vi "backup HPLC file.vi"(8 "error in (no error)":errorcluster, 10 "Backup location":path, 11 "HPLC":path) -> (0 "error out":errorcluster)   [LabVIEW 2017]
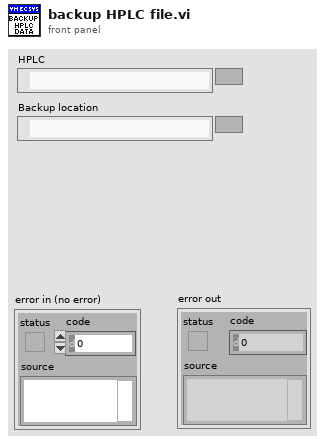
[diagram p1: front panel]
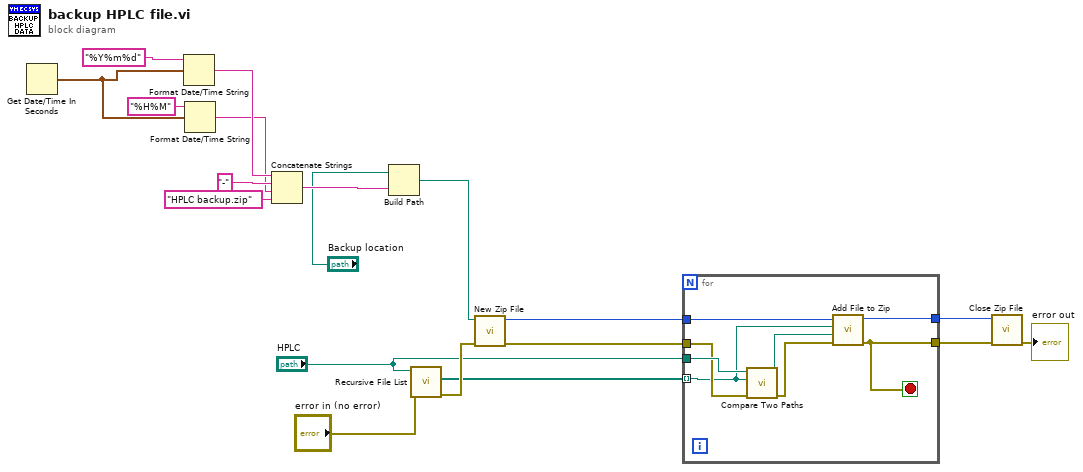
[diagram p0: block diagram]
diagram:
  n1 = Get Date/Time In Seconds() -> (seconds since 1Jan1904=w18:timestamp)
  n2 = Format Date/Time String(time format string (%c)="%Y%m%d", seconds (now)=w18) -> (date/time string=w16:string)  [unwired: 1 in]
  n3 = Format Date/Time String(time format string (%c)="%H%M", seconds (now)=w18) -> (date/time string=w14:string)  [unwired: 1 in]
  n4 = Concatenate Strings(w16, "-" ("string"), w14, "HPLC backup.zip" ("string")) -> (w13:string)
  n5 = Build Path(base path="Backup location", name or relative path=w13) -> (appended path=w1:path)
  n6 = call <vilib>:"Recursive File List.vi"("error in (no error)"="error in (no error)", "Folder Path"="HPLC") -> ("error out"=w12:errorcluster, "All Files in Dir"=w11:path[])  [unwired: 5 in, 3 out]
  n7 = call <vilib>:"New Zip File.vi"("error in (no error)"=w12, "target"=w1) -> ("error out"=w10:errorcluster, "zip file out"=w9:i64)  [unwired: 3 in, 1 out]
  n8 = for {
    tunnel: w11 -> [w23] mode=indexing
    tunnel: "HPLC" -> [w27]
    tunnel: w10 -> [w25]
    tunnel: w9 -> [w24]
    tunnel: [w21] -> w8
    tunnel: [w20] -> w7
    stop <- w20 stop-if-true
    n9 = call <vilib>:"Compare Two Paths.vi"("error in (no error)"=w25, "Path 2"=w23, "Path 1"=w27) -> ("error out"=w26:errorcluster, "Relative Path from 1 to 2"=w22:path)  [unwired: 5 in, 2 out]
    n10 = call <vilib>:"Add File to Zip.vi"("error in (no error)"=w26, "destination path in zip"=w22, "source file path"=w23, "zip file in"=w24) -> ("error out"=w20:errorcluster, "zip file out"=w21:i64)  [unwired: 6 in]
  }
  n11 = call <vilib>:"Close Zip File.vi"("error in (no error)"=w7, "zip file in"=w8) -> ("error out"=→"error out":errorcluster)  [unwired: 5 in]
